vi "MAIN_TDMS_save_path_definition.vi"(5 "error in":errorcluster, 8 "Path to the saving folder":path) -> (0 "error out":errorcluster, 3 "file or folder exists?":bool, 4 "path to tdms file":path)   [LabVIEW 2015]
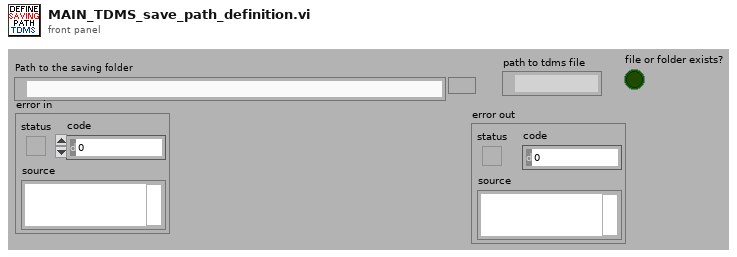
[diagram p1: front panel]
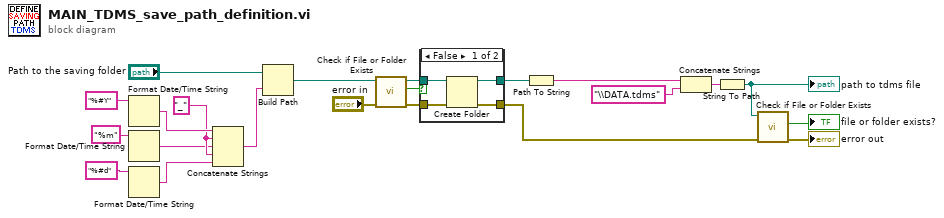
[diagram p0: block diagram]
diagram:
  w20 = "_" ("string")
  n1 = Format Date/Time String(time format string (%c)="%#Y") -> (date/time string=w21:string)  [unwired: 2 in]
  n2 = Format Date/Time String(time format string (%c)="%m") -> (date/time string=w17:string)  [unwired: 2 in]
  n3 = Format Date/Time String(time format string (%c)="%#d") -> (date/time string=w16:string)  [unwired: 2 in]
  n4 = Concatenate Strings(w21, w20, w17, w20, w16) -> (w14:string)
  n5 = Build Path(base path="Path to the saving folder", name or relative path=w14) -> (appended path=w13:path)
  n6 = call <vilib>:"Check if File or Folder Exists.vi"("error in (no error)"="error in", "path"=w13) -> ("error out"=w7:errorcluster, "file or folder exists?"=w6:bool, "dup path"=w8:path)  [unwired: 7 in]
  n7 = case shown="False" w6 {
    tunnel: w7 -> [w26 w27]
    tunnel: w8 -> [w25 w28]
    tunnel: [w24 w27] -> w1
    tunnel: [w23 w28] -> w2
    frame False {
      n8 = Create Folder(path (use dialog)=w25, error in=w26) -> (created path=w23:path, error out=w24:errorcluster)  [unwired: 1 in, 1 out]
    }
    frame True {
    }
  }
  n9 = Path To String(path=w2) -> (string=w11:string)
  n10 = Concatenate Strings(w11, "\\DATA.tdms" ("string")) -> (w9:string)
  n11 = String To Path(string=w9) -> (path=w5:path)
  "path to tdms file" <- w5
  n12 = call <vilib>:"Check if File or Folder Exists.vi"("error in (no error)"=w1, "path"=w5) -> ("error out"=→"error out":errorcluster, "file or folder exists?"=→"file or folder exists?":bool)  [unwired: 7 in, 1 out]
